vi "Untitled 1.vi"() -> ()   [LabVIEW 2012]
uses:
  InstrumentDll.dll
panel:
  out "return type 2":i32
  out "error out 2":errorcluster
  out "IQMeasRef":i32
  out "SpectrumMeasRef":i32
  out "rfsahandleout":i32
  out "return type":i32
  out "error out":errorcluster
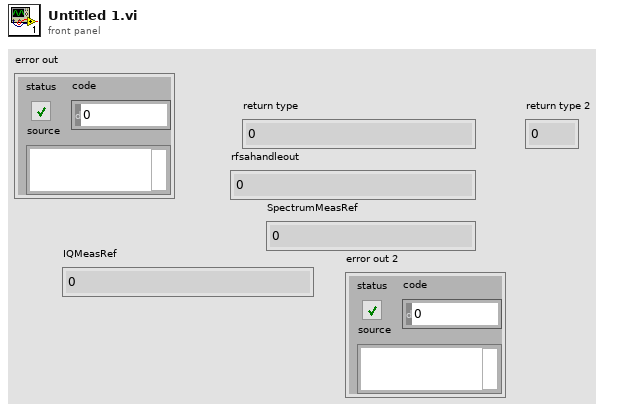
[diagram p1: front panel]
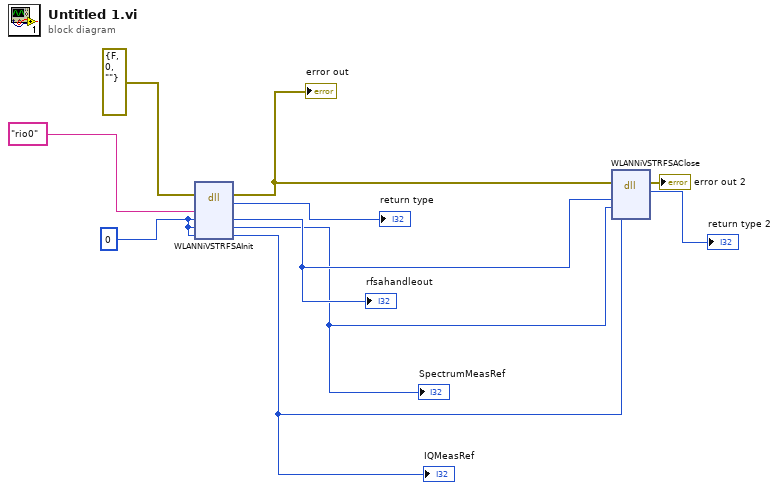
[diagram p0: block diagram]
diagram:
  w8 = 0 ("rfsahandleout")
  n1 = dll-call lib="C:/Users/ni/Desktop/NIVST for BBK/Wlan Instrument Code/BuildsDll/InstrumentDll.dll" fn="WLANNiVSTRFSAInit"(error in=errorcluster {"status"=FALSE, "code"=0, "source"=""} ("error in (no error)"), "rfsahandle"="rio0", "rfsahandleout"=w8, "SpectrumMeasRef"=w8, "IQMeasRef"=w8) -> (error out=w6:errorcluster, "return type"=→"return type":i32, "rfsahandleout"=w5:i32, "SpectrumMeasRef"=w4:i32, "IQMeasRef"=w3:i32)  [unwired: 3 in, 1 out]
  "error out" <- w6
  "rfsahandleout" <- w5
  "SpectrumMeasRef" <- w4
  "IQMeasRef" <- w3
  n2 = dll-call lib="C:/Users/ni/Desktop/NIVST for BBK/Wlan Instrument Code/BuildsDll/InstrumentDll.dll" fn="WLANNiVSTRFSAClose"(error in=w6, "rfsahandleout"=w5, "SpectrumMeasRef"=w4, "IQMeasRef"=w3) -> (error out=→"error out 2":errorcluster, "return type"=→"return type 2":i32)  [unwired: 5 in, 1 out]
